vi "Constantes.vi"() -> ()   [LabVIEW 2016]
panel:
  in  "Joystick DeadZone":dbl(slide) scale=0.0..1.0
  in  "Input Y Factor":dbl(slide) scale=0.0..1.0
  in  "Input X Factor":dbl(slide) scale=0.0..1.0
  in  "Block forward when distance to a wall is under":dbl
  # "Teleop Driving"
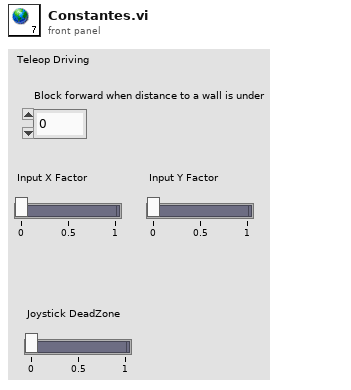
[diagram p1: front panel]
diagram:
